vi "题目五.vi"() -> ()   [LabVIEW 2017]
panel:
  out "日期/时间字符串":string
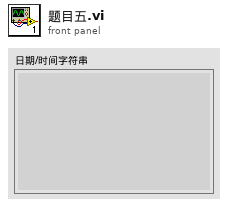
[diagram p1: front panel]
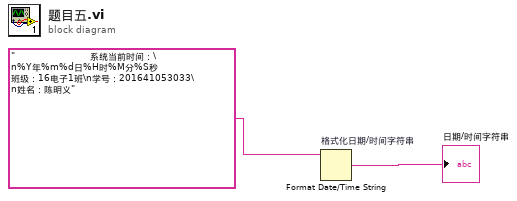
[diagram p0: block diagram]
diagram:
  n1 = Format Date/Time String "格式化日期/时间字符串"(time format string (%c)="                         系统当前时间：\n%Y年%m%d日%H时%M分%S秒                        班级：16电子1班\n学号：201641053033\n姓名：陈明义") -> (date/time string=→"日期/时间字符串":string)  [unwired: 2 in]
